vi "Write Grayscale Image.vi"(8 "error in (no error)":errorcluster, 10 "Image":T1, 11 "Video Frame in":refnum<class "Video Frame.lvclass">) -> (0 "error out":errorcluster, 3 "Video Frame out":refnum<class "Video Frame.lvclass">)   [LabVIEW 2018, in "Video Frame.lvclass"]
uses:
  Video Frame.lvclass
  <vilib>/vision/Image Controls.llb/IMAQ Image.ctl
  Video Frame.lvclass/Video Frame.ctl
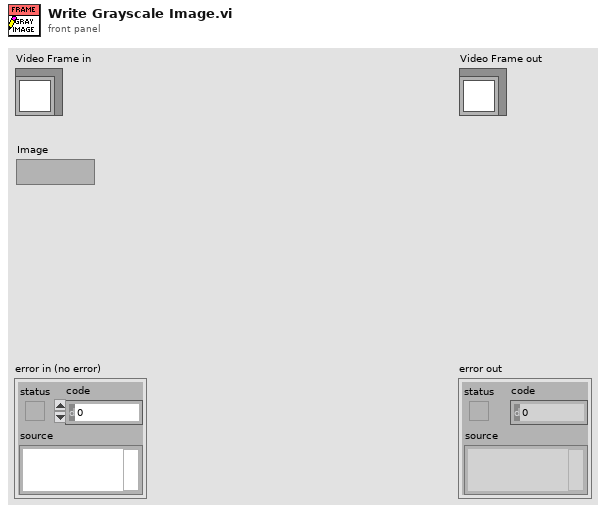
[diagram p1: front panel]
types:
  T1 = typedef "IMAQ Image.ctl" = refnum<image>
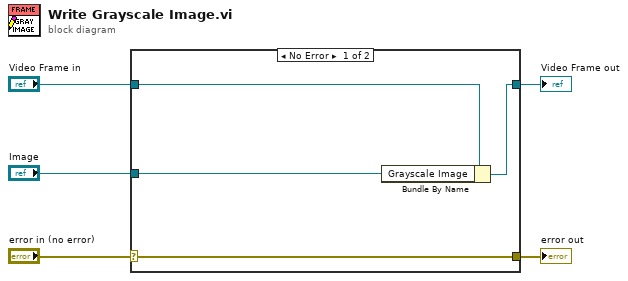
[diagram p0: block diagram]
diagram:
  n1 = case shown="No Error" "error in (no error)" {
    selector: "error in (no error)" -> [w9 w10]
    tunnel: [w9 w10] -> w4
    tunnel: [w7 w11] -> w2
    tunnel: "Video Frame in" -> [w8 w11]
    tunnel: "Image" -> [w6 _]
    frame No Error {
      n2 = Bundle By Name(cluster=w8, "Grayscale Image"=w6) -> (w7:refnum<class "Video Frame.lvclass">)
    }
    frame Error {
    }
  }
  "error out" <- w4
  "Video Frame out" <- w2
